vi "Test Discovery Listener.vi"() -> ()   [LabVIEW 2020]
uses:
  Source/Public/Discovery/Typedefs/Server Beacon.ctl
panel:
  out "Beacon":T1={"name"="", "addr"="", "port"=0, "ver"=10001}
  in  "stop":bool
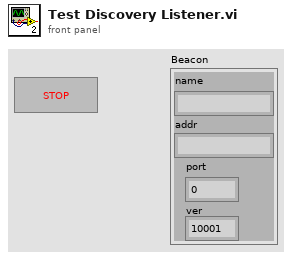
[diagram p1: front panel]
types:
  T1 = typedef "Server Beacon.ctl" = cluster{"name":string, "addr":string, "port":u16, "ver":u16}
  T2 = cluster{"DiscoveredHost":refnum<user-event>, "ExpiredHost":refnum<user-event>}
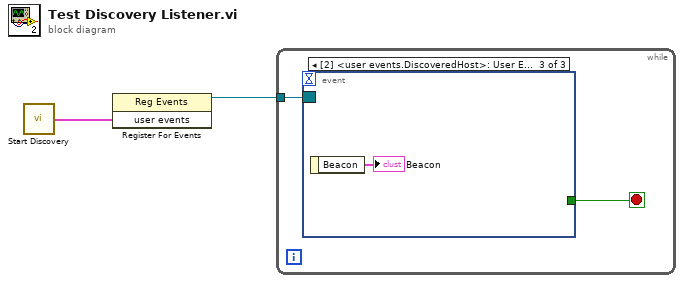
[diagram p0: block diagram]
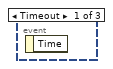
[diagram p2: hidden frame]
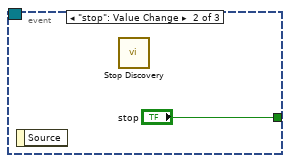
[diagram p3: hidden frame]
diagram:
  n1 = call "Start Discovery.vi"() -> ("user events"=w2:T2)  [unwired: 14 in, 1 out]
  n2 = register-events(w2) -> (reference out=w1:refnum<event-registration>)  [unwired: 2 in, 1 out]
  n3 = while {
    tunnel: w1 -> [w4]
    stop <- w3 stop-if-true
    n4 = event shown="[2] <user events.DiscoveredHost>: User Event" {
      selector: w4 -> [_ _ _]
      dyn-events: _ -> [_ _ _]
      timeout: _ -> [_ _ _]
      tunnel: [_ "stop" _] -> w3
      event Timeout {
        n5 = event-data() -> ()  [unwired: 1 in, 1 out]
      }
      event "stop": Value Change {
        n6 = event-data() -> ()  [unwired: 1 in, 1 out]
        n7 = call "Stop Discovery.vi"() -> ()  [unwired: 12 in]
      }
      event User Event {
        n8 = event-data() -> ("Beacon"=→"Beacon":T1)  [unwired: 1 in]
      }
    }
  }
